vi "Set Name and Library.vi"(8 "error in (no error)":errorcluster, 10 "Top-Level Library Ref":refnum<vi>, 11 "NI_AB_API_PPL in":refnum<class "NI_AB_API_PPL.lvclass">) -> (0 "error out":errorcluster, 2 "PPL Name":string, 3 "NI_AB_API_PPL out":refnum<class "NI_AB_API_PPL.lvclass">)   [LabVIEW 2019]
uses:
  <vilib>/AppBuilder/AB_API/PPL/NI_AB_API_PPL.lvclass
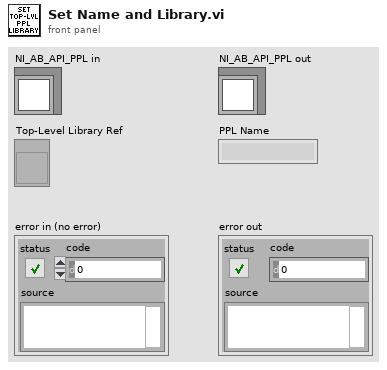
[diagram p1: front panel]
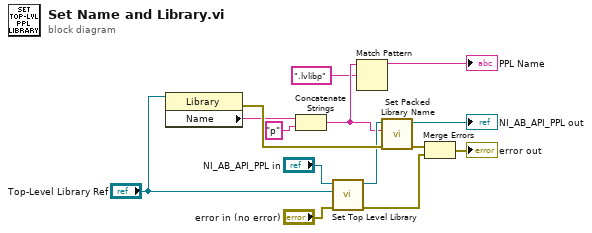
[diagram p0: block diagram]
diagram:
  n1 = property class="Library"(reference="Top-Level Library Ref") -> (error out=w14:errorcluster, "Name"=w10:string)  [unwired: 1 in, 1 out]
  n2 = Concatenate Strings(w10, "p" ("string")) -> (w4:string)
  n3 = call-dynamic "Set Top Level Library.vi"("error in (no error)"="error in (no error)", "ProjectItem Refnum"="Top-Level Library Ref", "PPL in"="NI_AB_API_PPL in") -> ("error out"=w1:errorcluster, "PPL out"=w12:refnum<class "NI_AB_API_PPL.lvclass">)  [unwired: 7 in]
  n4 = Match Pattern(string=w4, regular expression=".lvlibp") -> (before substring=→"PPL Name":string)  [unwired: 1 in, 3 out]
  n5 = call-dynamic "Set Packed Library Name.vi"("error in (no error)"=w14, "Packed library name"=w4, "PPL in"=w12) -> ("error out"=w5:errorcluster, "PPL out"=→"NI_AB_API_PPL out":refnum<class "NI_AB_API_PPL.lvclass">)  [unwired: 7 in]
  n6 = Merge Errors(w5, w1) -> (→"error out":errorcluster)
